vi "A_D_Reading.vi"(8 "error in (no error)":errorcluster, 10 "A/D Channel":dbl, 11 "SRV In":refnum<k5>) -> (0 "error out":errorcluster, 1 "Reply":string, 2 "A/D Value":i32, 3 "SRV Out":refnum<k5>)   [LabVIEW 2009]
doc: "Request and read A/D values from the SRV.\n\n\nWritten for Benilde St. Margaret's School - Tim Jump\nBy Doug Schmertman - Logic PD\nCopyright 2012"
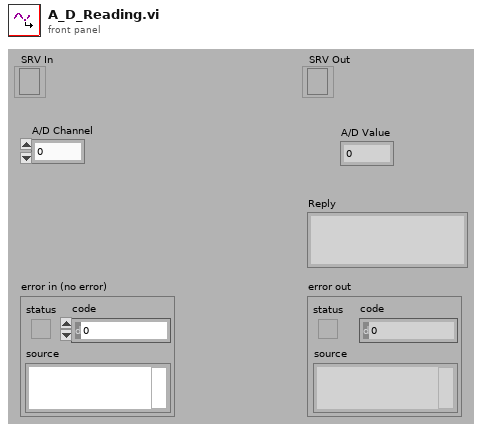
[diagram p1: front panel]
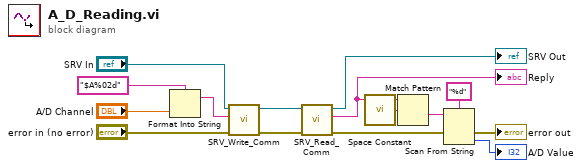
[diagram p0: block diagram]
diagram:
  n1 = Format Into String(format string="$A%02d" ("Command Sent"), "A/D Channel") -> (resulting string=w10:string)  [unwired: 2 in, 1 out]
  n2 = call "SRV_Write_Comm.vi"("error in (no error)"="error in (no error)", "Command Sent"=w10, "SRV In"="SRV In") -> ("error out"=w9:errorcluster, "SRV Out"=w8:refnum<k5>)  [unwired: 6 in, 1 out]
  n3 = call "SRV_Read_Comm.vi"("error in (no error)"=w9, "SRV In"=w8) -> ("error out"=w2:errorcluster, "Data out"=w3:string, "SRV Out"=→"SRV Out":refnum<k5>)  [unwired: 7 in]
  "Reply" <- w3
  n4 = call <vilib>:"Space Constant.vi"() -> ("String"=w6:string)
  n5 = Match Pattern(string=w3, regular expression=w6) -> (after substring=w5:string)  [unwired: 1 in, 3 out]
  n6 = Scan From String(format string="%d", input string=w5, error in=w2) -> (error out=→"error out":errorcluster, output 1=→"A/D Value":i32)  [unwired: 2 in, 2 out]
